vi "Load and Vin SMU Measurement.vi"() -> ()   [LabVIEW 2021]
doc: "Demonstrates how to use the DC Voltage Output Function to force an output voltage. This example initializes a session, configures the Output Function, Sense, Autorange, Voltage Level and Current Limit, initiates generation, waits for a specified delay, and measures the voltage and current output. This example uses Single Point source mode."
uses:
  <instrlib>/niDCPower/nidcpower.llb/niDCPower Output Function.ctl
  <instrlib>/niDCPower/nidcpower.llb/niDCPower Source Mode.ctl
panel:
  in  "Load SMU":refnum<k15>="Dev1"
  in  "Load SMU Channel":string="0"
  in  "Current Level":dbl=0.01 format="%.3p"
  in  "Voltage Limit":dbl=2.0 format="%.5p"
  out "Load SMU Current":dbl
  out "Load SMU Voltage":dbl
  in  "error in":errorcluster
  out "error out":errorcluster
  out "Voltage Measurement":dbl caption="Vin SMU Voltage"
  out "Current Measurement":dbl caption="Vin SMU Current"
  in  "Current Limit":dbl=0.01 format="%.3p"
  in  "Voltage Level":dbl=2.0 format="%.5p"
  in  "Vin SMU Channel":string="0"
  in  "Vin SMU":refnum<k15>="Dev1"
  # "Overview: Demonstrates how to use the DC Voltage Output Function to force an output voltage.  \nThis example initializes a session; configures the Output Function, Voltage Level and Current Limit; \ninitiates generation; waits for a specified delay; and measures the voltage and current output. \nRequirements: NI-DCPower\nInstructions:\n1. Select the appropriate device in the Resource Name control.\n2. Configure the parameters of the DC Voltage signal you'd like to output.\n3. Run the VI."
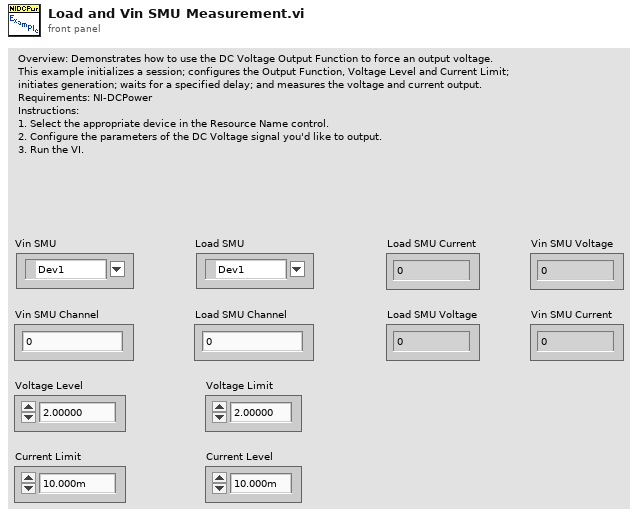
[diagram p1: front panel]
types:
  T1 = typedef "niDCPower Output Function.ctl" = i32
  T2 = typedef "niDCPower Source Mode.ctl" = i32
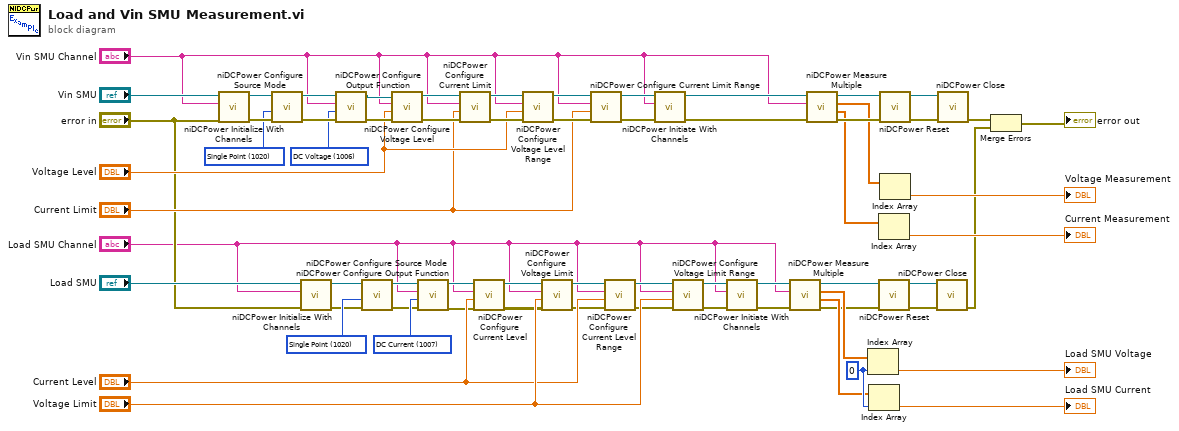
[diagram p0: block diagram]
diagram:
  w33 = T1 1007 items=["DC Voltage"=1006, "DC Current"=1007, "Pulse Voltage"=1049, "Pulse Current"=1050] ("output function")
  w24 = 0 ("index")
  w15 = T2 1020 items=["Single Point"=1020, "Sequence"=1021] ("source mode")
  w43 = T1 1006 items=["DC Voltage"=1006, "DC Current"=1007, "Pulse Voltage"=1049, "Pulse Current"=1050] ("output function")
  w56 = T2 1020 items=["Single Point"=1020, "Sequence"=1021] ("source mode")
  n1 = call <instrlib>:"niDCPower Initialize With Channels.vi"("error in (no error)"="error in", "channels"="Vin SMU Channel", "resource name"="Vin SMU") -> ("error out"=w60:errorcluster, "instrument handle out"=w59:refnum<k15>)  [unwired: 2 in, 5 out]
  n2 = call <instrlib>:"niDCPower Configure Source Mode.vi"("error in (no error)"=w60, "source mode"=w56, "instrument handle"=w59) -> ("error out"=w58:errorcluster, "instrument handle out"=w57:refnum<k15>)  [unwired: 7 out]
  n3 = call <instrlib>:"niDCPower Initialize With Channels.vi"("error in (no error)"="error in", "channels"="Load SMU Channel", "resource name"="Load SMU") -> ("error out"=w11:errorcluster, "instrument handle out"=w12:refnum<k15>)  [unwired: 2 in, 5 out]
  n4 = call <instrlib>:"niDCPower Configure Output Function.vi"("error in (no error)"=w58, "output function"=w43, "channel name"="Vin SMU Channel", "instrument handle"=w57) -> ("error out"=w44:errorcluster, "instrument handle out"=w45:refnum<k15>)  [unwired: 6 out]
  n5 = call <instrlib>:"niDCPower Configure Source Mode.vi"("error in (no error)"=w11, "source mode"=w15, "instrument handle"=w12) -> ("error out"=w13:errorcluster, "instrument handle out"=w14:refnum<k15>)  [unwired: 7 out]
  n6 = call <instrlib>:"niDCPower Configure Voltage Level.vi"("error in (no error)"=w44, "voltage level"="Voltage Level", "channel name"="Vin SMU Channel", "instrument handle"=w45) -> ("error out"=w63:errorcluster, "instrument handle out"=w64:refnum<k15>)  [unwired: 6 out]
  n7 = call <instrlib>:"niDCPower Configure Output Function.vi"("error in (no error)"=w13, "output function"=w33, "channel name"="Load SMU Channel", "instrument handle"=w14) -> ("error out"=w31:errorcluster, "instrument handle out"=w32:refnum<k15>)  [unwired: 6 out]
  n8 = call <instrlib>:"niDCPower Configure Current Limit.vi"("error in (no error)"=w63, "current limit"="Current Limit", "channel name"="Vin SMU Channel", "instrument handle"=w64) -> ("error out"=w55:errorcluster, "instrument handle out"=w54:refnum<k15>)  [unwired: 1 in, 5 out]
  n9 = call <instrlib>:"niDCPower Configure Current Level.vi"("error in (no error)"=w31, "current level"="Current Level", "channel name"="Load SMU Channel", "instrument handle"=w32) -> ("error out"=w8:errorcluster, "instrument handle out"=w7:refnum<k15>)  [unwired: 6 out]
  n10 = call <instrlib>:"niDCPower Configure Voltage Level Range.vi"("error in (no error)"=w55, "voltage level range"="Voltage Level", "channel name"="Vin SMU Channel", "instrument handle"=w54) -> ("error out"=w53:errorcluster, "instrument handle out"=w52:refnum<k15>)  [unwired: 6 out]
  n11 = call <instrlib>:"niDCPower Configure Voltage Limit.vi"("error in (no error)"=w8, "voltage limit"="Voltage Limit", "channel name"="Load SMU Channel", "instrument handle"=w7) -> ("error out"=w16:errorcluster, "instrument handle out"=w17:refnum<k15>)  [unwired: 6 out]
  n12 = call <instrlib>:"niDCPower Configure Current Limit Range.vi"("error in (no error)"=w53, "current limit range"="Current Limit", "channel name"="Vin SMU Channel", "instrument handle"=w52) -> ("error out"=w48:errorcluster, "instrument handle out"=w49:refnum<k15>)  [unwired: 6 out]
  n13 = call <instrlib>:"niDCPower Configure Current Level Range.vi"("error in (no error)"=w16, "current level range"="Current Level", "channel name"="Load SMU Channel", "instrument handle"=w17) -> ("error out"=w18:errorcluster, "instrument handle out"=w19:refnum<k15>)  [unwired: 6 out]
  n14 = call <instrlib>:"niDCPower Initiate With Channels.vi"("error in (no error)"=w48, "channel name"="Vin SMU Channel", "instrument handle"=w49) -> ("error out"=w46:errorcluster, "instrument handle out"=w47:refnum<k15>)  [unwired: 7 in]
  n15 = call <instrlib>:"niDCPower Configure Voltage Limit Range.vi"("error in (no error)"=w18, "voltage limit range"="Voltage Limit", "channel name"="Load SMU Channel", "instrument handle"=w19) -> ("error out"=w28:errorcluster, "instrument handle out"=w27:refnum<k15>)  [unwired: 6 out]
  n16 = call <instrlib>:"niDCPower Initiate With Channels.vi"("error in (no error)"=w28, "channel name"="Load SMU Channel", "instrument handle"=w27) -> ("error out"=w30:errorcluster, "instrument handle out"=w29:refnum<k15>)  [unwired: 7 in]
  n17 = call <instrlib>:"niDCPower Measure Multiple.vi"("error in (no error)"=w30, "channel name"="Load SMU Channel", "instrument handle"=w29) -> ("error out"=w21:errorcluster, "current measurements"=w23:dbl[], "voltage measurements"=w22:dbl[], "instrument handle out"=w20:refnum<k15>)  [unwired: 5 out]
  n18 = call <instrlib>:"niDCPower Measure Multiple.vi"("error in (no error)"=w46, "channel name"="Vin SMU Channel", "instrument handle"=w47) -> ("error out"=w50:errorcluster, "current measurements"=w41:dbl[], "voltage measurements"=w39:dbl[], "instrument handle out"=w51:refnum<k15>)  [unwired: 5 out]
  n19 = Index Array(array=w22, index=w24) -> (element=→"Load SMU Voltage":dbl)
  n20 = Index Array(array=w23, index=w24) -> (element=→"Load SMU Current":dbl)
  n21 = Index Array(array=w41) -> (element=→"Current Measurement":dbl)  [unwired: 1 in]
  n22 = call <instrlib>:"niDCPower Reset.vi"("error in (no error)"=w21, "instrument handle"=w20) -> ("error out"=w10:errorcluster, "instrument handle out"=w9:refnum<k15>)  [unwired: 2 in, 6 out]
  n23 = call <instrlib>:"niDCPower Reset.vi"("error in (no error)"=w50, "instrument handle"=w51) -> ("error out"=w61:errorcluster, "instrument handle out"=w62:refnum<k15>)  [unwired: 2 in, 6 out]
  n24 = Index Array(array=w39) -> (element=→"Voltage Measurement":dbl)  [unwired: 1 in]
  n25 = call <instrlib>:"niDCPower Close.vi"("error in (no error)"=w10, "instrument handle"=w9) -> ("error out"=w3:errorcluster)  [unwired: 9 out]
  n26 = call <instrlib>:"niDCPower Close.vi"("error in (no error)"=w61, "instrument handle"=w62) -> ("error out"=w42:errorcluster)  [unwired: 9 out]
  n27 = Merge Errors(w42, w3) -> (→"error out":errorcluster)
